vi "ErrorDefinitionSQLite_Create.vi"(8 "ErrorIn":errorcluster caption="Error In(no Error)", 11 "ReferenceIn":refnum<class "ErrorDefinitionSQLite.lvclass"> caption="Reference In") -> (0 "ErrorOut":errorcluster caption="Error Out", 3 "ReferenceOut":refnum<class "ErrorDefinitionSQLite.lvclass"> caption="Reference Out")   [LabVIEW 2021, in "ErrorDefinitionSQLite.lvclass"]
uses:
  ErrorDefinitionSQLite.lvclass
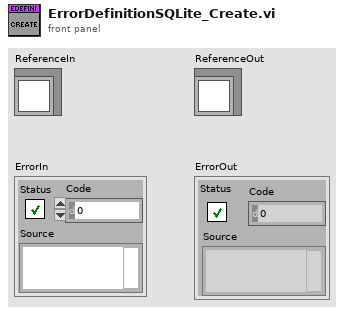
[diagram p1: front panel]
types:
  T1 = typedef "ErrorDefinitionSQLite.lvclass/ObjectAttributes.ctl" = cluster{"Path":path, "SQLiteRef":refnum<class "Connection.lvclass">, "EndOfRange":i32, "StartOfRange":i32}
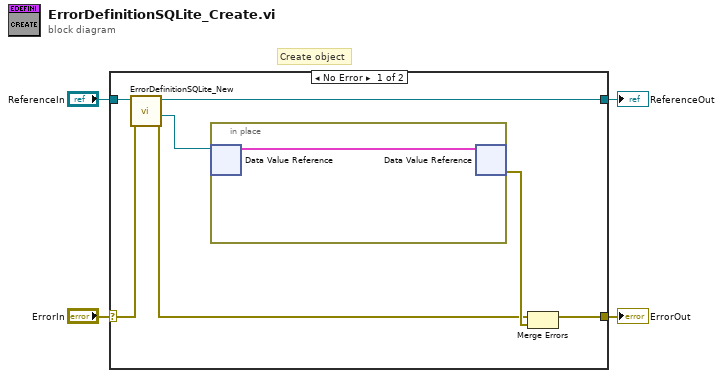
[diagram p0: block diagram]
diagram:
  # "Create object"
  n1 = case shown="No Error" "ErrorIn" {
    selector: "ErrorIn" -> [w11 w14]
    tunnel: [w9 w14] -> w3
    tunnel: "ReferenceIn" -> [w7 w13]
    tunnel: [w6 w13] -> w1
    frame No Error {
      n2 = call "ErrorDefinitionSQLite_New.vi"("ErrorIn"=w11, "ReferenceIn"=w7) -> ("ErrorOut"=w8:errorcluster, "DVRRefOut"=w5:refnum<data-value>, "ReferenceOut"=w6:refnum<class "ErrorDefinitionSQLite.lvclass">)  [unwired: 6 in, 1 out]
      n3 = in-place "In Place Element Structure" {
        n4 = in-place-dvr #1(w5) -> (w12:T1)  [unwired: 1 out]
        n5 = in-place-dvr #1(w12) -> (w10:errorcluster)  [unwired: 1 out]
      }
      n6 = Merge Errors(w8, w10) -> (w9:errorcluster)
    }
    frame Error {
    }
  }
  "ErrorOut" <- w3
  "ReferenceOut" <- w1
